vi "VI_GetELOGChNames.vi"(8 "error in (no error)":errorcluster, 11 "Common Refs":T1={"LBox_ChList"=refnum, "STR_LoggingChName1"=refnum, "Listbox_ChValue"=refnum, "STR_LoggingChName2"=refnum, "STR_LoggingChName3"=refnum, "STR_LoggingChName4"=refnum, "STR_LoggingChName5"=refnum, "STR_LoggingChName6"=refnum, "OXY_SCPI Ref"="TCPIP0::192.168.1.75::10001::SOCKET", "STR_ChName1"=refnum, "STR_ChName2"=refnum, "STR_ChName3"=refnum, "STR_ChName4"=refnum, "STR_ChName5"=refnum, "STR_ChName6"=refnum, "Enum_SelectTimestampFormat"=refnum, "GRAPH-XY_ELOG"=refnum, "GRAPH-XY_Measurement"=refnum, "Button_StartBuffer"=refnum, "Button_StopBuffer"=refnum, "Button_FetchData"=refnum, "STR_LoggingChName1"=refnum, "STR_LoggingChName2"=refnum, "STR_LoggingChName3"=refnum, "STR_LoggingChName4"=refnum, "STR_LoggingChName5"=refnum, "STR_LoggingChName6"=refnum, "Enum_SelectCalc"=refnum, "Num_SetDurationTime"=refnum, "Button_StopTransfer"=refnum, "Button_StartTransfer"=refnum, "STR_IN_AggregationRate"=refnum, "Button_Disconnect"=refnum, "Button_Connect"=refnum, "Button_StartRec"=refnum, "Button_PauseRec"=refnum, "Button_StopRec"=refnum, "Bool_StatusLED"=refnum, "Indicator_RecordingStatus"=refnum}) -> (0 "error out":errorcluster, 2 "ChNames (Array)":string[](array[string]), 3 "ChNames (Single String)":string)   [LabVIEW 2018]
uses:
  TypeDefs/Refs_Common.ctl
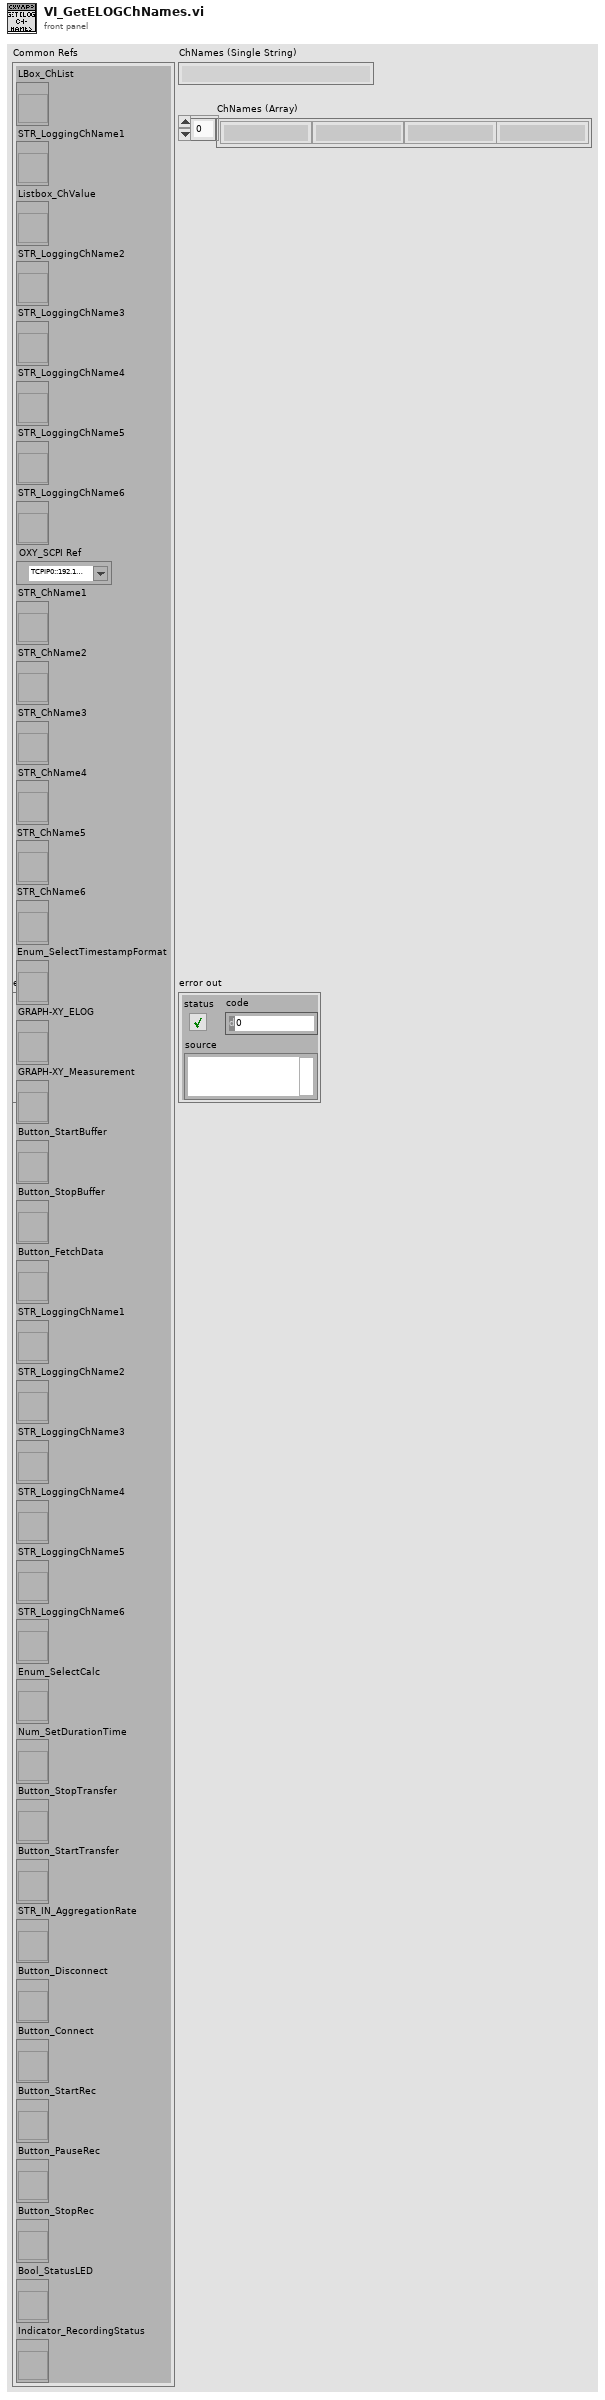
[diagram p1: front panel]
types:
  T1 = typedef "Refs_Common.ctl" = cluster{"LBox_ChList":refnum<vi>, "STR_LoggingChName1":refnum<vi>, "Listbox_ChValue":refnum<vi>, "STR_LoggingChName2":refnum<vi>, "STR_LoggingChName3":refnum<vi>, "STR_LoggingChName4":refnum<vi>, "STR_LoggingChName5":refnum<vi>, "STR_LoggingChName6":refnum<vi>, "OXY_SCPI Ref":refnum<visa-resource-name>, "STR_ChName1":refnum<vi>, "STR_ChName2":refnum<vi>, "STR_ChName3":refnum<vi>, "STR_ChName4":refnum<vi>, "STR_ChName5":refnum<vi>, "STR_ChName6":refnum<vi>, "Enum_SelectTimestampFormat":refnum<vi>, "GRAPH-XY_ELOG":refnum<vi>, "GRAPH-XY_Measurement":refnum<vi>, "Button_StartBuffer":refnum<vi>, "Button_StopBuffer":refnum<vi>, "Button_FetchData":refnum<vi>, "STR_LoggingChName1":refnum<vi>, "STR_LoggingChName2":refnum<vi>, "STR_LoggingChName3":refnum<vi>, "STR_LoggingChName4":refnum<vi>, "STR_LoggingChName5":refnum<vi>, "STR_LoggingChName6":refnum<vi>, "Enum_SelectCalc":refnum<vi>, "Num_SetDurationTime":refnum<vi>, "Button_StopTransfer":refnum<vi>, "Button_StartTransfer":refnum<vi>, "STR_IN_AggregationRate":refnum<vi>, "Button_Disconnect":refnum<vi>, "Button_Connect":refnum<vi>, "Button_StartRec":refnum<vi>, "Button_PauseRec":refnum<vi>, "Button_StopRec":refnum<vi>, "Bool_StatusLED":refnum<vi>, "Indicator_RecordingStatus":refnum<vi>}
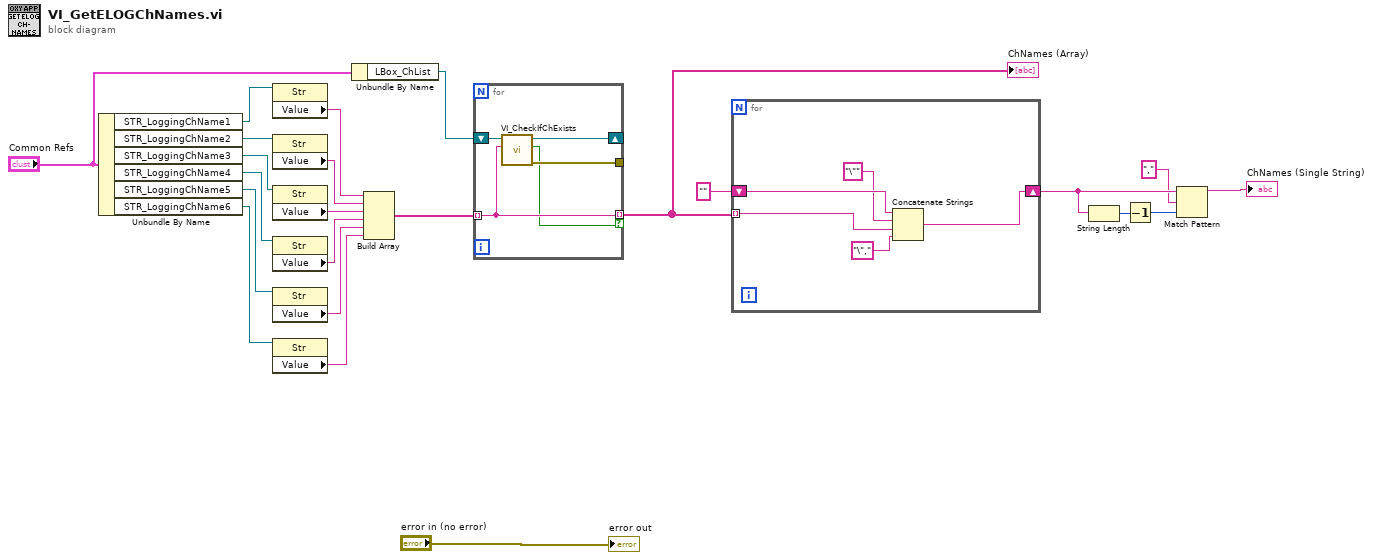
[diagram p0: block diagram]
diagram:
  n1 = Unbundle By Name("Common Refs") -> ("STR_LoggingChName1"=w12:refnum<vi>, "STR_LoggingChName2"=w11:refnum<vi>, "STR_LoggingChName3"=w10:refnum<vi>, "STR_LoggingChName4"=w9:refnum<vi>, "STR_LoggingChName5"=w8:refnum<vi>, "STR_LoggingChName6"=w7:refnum<vi>)
  n2 = property class="Str"(reference=w12) -> ("Value"=w6:string)  [unwired: 1 in, 2 out]
  n3 = property class="Str"(reference=w11) -> ("Value"=w5:string)  [unwired: 1 in, 2 out]
  n4 = property class="Str"(reference=w10) -> ("Value"=w4:string)  [unwired: 1 in, 2 out]
  n5 = property class="Str"(reference=w9) -> ("Value"=w3:string)  [unwired: 1 in, 2 out]
  n6 = property class="Str"(reference=w8) -> ("Value"=w2:string)  [unwired: 1 in, 2 out]
  n7 = property class="Str"(reference=w7) -> ("Value"=w1:string)  [unwired: 1 in, 2 out]
  n8 = Unbundle By Name("Common Refs") -> ("LBox_ChList"=w13:refnum<vi>)
  n9 = Build Array(w6, w5, w4, w3, w2, w1) -> (w14:string[])
  n10 = for {
    tunnel: w14 -> [w25] mode=indexing
    shift-right: [w27] -> _
    shift-left: w13 -> [w28]
    tunnel: [w26] -> _
    tunnel: [w25] -> w22 mode=indexing if=w24
    n11 = call "VI_CheckIfChExists.vi"("Channel Name To Check"=w25, "ChList_Ref In"=w28) -> ("error out"=w26:errorcluster, "Channel Exists"=w24:bool, "ChList_Ref Out"=w27:refnum<vi>)  [unwired: 7 in]
  }
  "ChNames (Array)" <- w22
  n12 = for {
    tunnel: w22 -> [w30] mode=indexing
    shift-right: [w32] -> w19
    shift-left: "" ("f") -> [w33]
    n13 = Concatenate Strings(w33, "\"" ("string"), w30, "\"," ("string")) -> (w32:string)
  }
  n14 = String Length(string=w19) -> (length=w20:i32)
  n15 = Decrement(x=w20) -> (x-1=w18:i32)
  n16 = Match Pattern(string=w19, regular expression=",", offset (0)=w18) -> (before substring=→"ChNames (Single String)":string)  [unwired: 3 out]
  "error out" <- "error in (no error)"
